vi "boxcar_smoothing_DV.vi"(0 "iteration Number":i32=2, 2 "smooth factor":i32=121, 3 "raw data":dbl[](array[numeric]) format="%.2e") -> (1 "smoothed":dbl[](array[numeric]) format="%.3e")   [LabVIEW 2020]
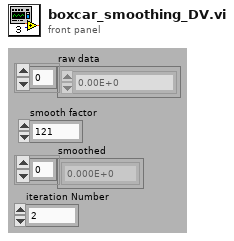
[diagram p1: front panel]
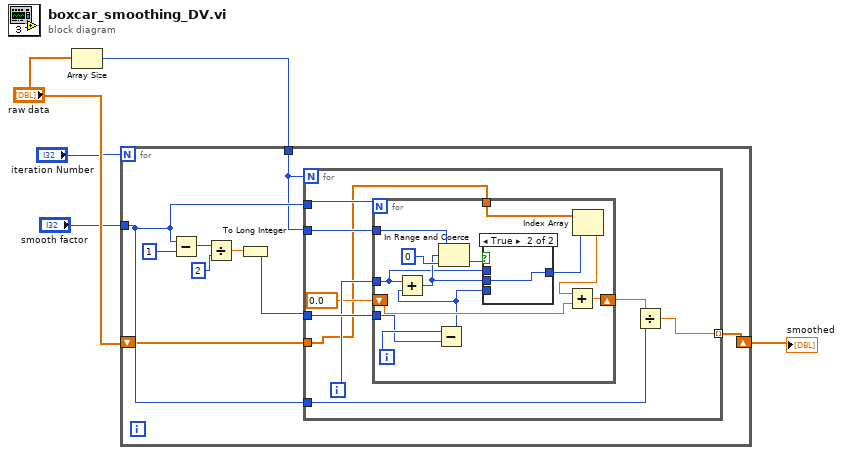
[diagram p0: block diagram]
diagram:
  n1 = Array Size(array="raw data") -> (size(s)=w3:i32)
  n2 = for {
    N: "iteration Number" -> [_]
    tunnel: "smooth factor" -> [w10]
    tunnel: w3 -> [w8]
    shift-right: [w6] -> w2
    shift-left: "raw data" -> [w7]
    n3 = Subtract(x=w10, y=1) -> (x-y=w12:i32)
    n4 = Divide(x=w12, y=2) -> (x/y=w14:dbl)
    n5 = To Long Integer(number=w14) -> (32bit integer=w9:i32)
    n6 = for {
      N: w8 -> [_]
      tunnel: w9 -> [w23]
      tunnel: w8 -> [w19]
      tunnel: w10 -> [w18]
      tunnel: w10 -> [w17]
      tunnel: w7 -> [w16]
      tunnel: [w15] -> w6 mode=indexing
      i -> [w22]
      n7 = for {
        N: w18 -> [_]
        tunnel: w23 -> [w35]
        tunnel: w22 -> [w26]
        shift-right: [w32] -> w20
        shift-left: 0.0 -> [w33]
        tunnel: w19 -> [w31]
        tunnel: w16 -> [w24]
        i -> [w36]
        n8 = Subtract(x=w36, y=w35) -> (x-y=w25:i32)
        n9 = Add(x=w26, y=w25) -> (x+y=w27:i32)
        n10 = In Range and Coerce(upper limit=w31, x=w27, lower limit=u8 0) -> (In Range?=w29:bool)  [unwired: 1 out]
        n11 = case shown="True" w29 {
          tunnel: [w37 w38] -> w28
          tunnel: w27 -> [_ w38]
          tunnel: w26 -> [w37 _]
          tunnel: w25 -> [_ _]
          frame False {
          }
          frame True {
          }
        }
        n12 = Index Array(array=w24, index=w28) -> (element=w34:dbl)
        n13 = Add(x=w34, y=w33) -> (x+y=w32:dbl)
      }
      n14 = Divide(x=w20, y=w17) -> (x/y=w15:dbl)
    }
  }
  "smoothed" <- w2
